vi "FPGA.vi"() -> ()   [LabVIEW 2016]
doc: "FPGA.vi\nv4.0c\nBuggy competition FPGA\n\nA Jackson 01/01/14"
uses:
  <vilib>/rvi/Emulation/niFpgaGetClockAttributes.vi
  <vilib>/rvi/Emulation/niFpgaSctlEmulationGetInTimedLoop.vi
  <vilib>/rvi/Emulation/niFpgaEmulationReportErrorSimple.vi
  <vilib>/rvi/Emulation/niFpgaProcessEmulError.vi
  <vilib>/rvi/eio/common/nirviEmuTemplateMethod_errors.vi
  <vilib>/rvi/Emulation/niFpgaCriticalErrorInLSC.vi
  <vilib>/eio/EIONode/EIONode.xnode
panel:
  in  "MS3":bool
  in  "MS2":bool
  in  "MS1":bool
  out "Motors Enabled":bool=TRUE
  in  "Motor 2 command":i8
  in  "Motor 1 command":i8
  out "Motor 2 Steps":i16
  out "Motor 1 Steps":i16
  in  "Motor Enable":bool
  in  "Step time":u32=100
  out "Potentiometer (V)":i16
  in  "Max sample interval (uS)":u32=62500
  in  "Measurement Width (Counts)":i64=4
  out "Enc 2 Interval (uS)":u32=10000000
  out "Enc 1 Interval (uS)":u32=10000000
  out "Encoder 2 dt (uS)":i64=-41
  out "Encoder 1 dt (uS)":i64=-41
  in  "Loop dT (uS)":u32=20
  out "Act. Loop uS":u32=20
  in  "Filter Iterations":i16=2
  in  "Reset encoder 1":bool
  out "Loop Count":i32=24102111
  out "Switch B (Blue)":bool
  out "Switch A (Green)":bool
  out "Encoder 2 Count":i64=-1
  out "Encoder 1 Count":i64=-1
  in  "Reset encoder 2":bool
  in  "stop":bool
  # "This FPGA VI will be controlled by the real-time VI and carries out low level hardware\n I/O via the FPGA part of the cRIO but it can also be used as a test panel for plotter hardware."
  # "Motors"
  # "Encoders"
  # "Timing"
  # "Microstepping"
  # "Switches"
  # "Potentiometer"
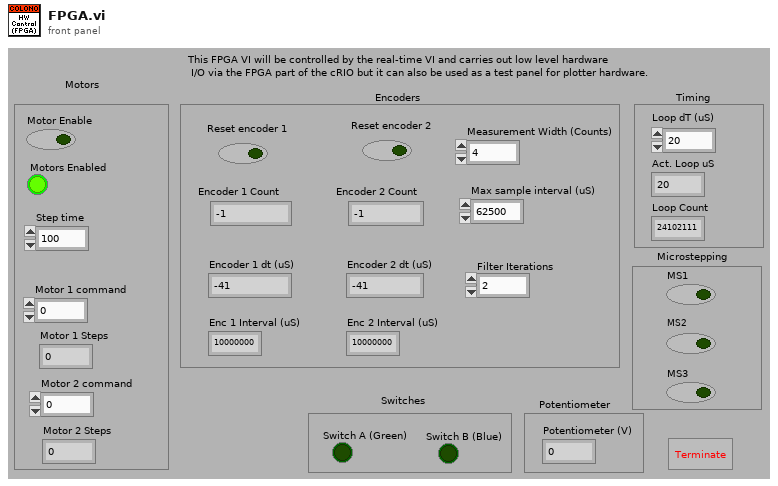
[diagram p1: front panel]
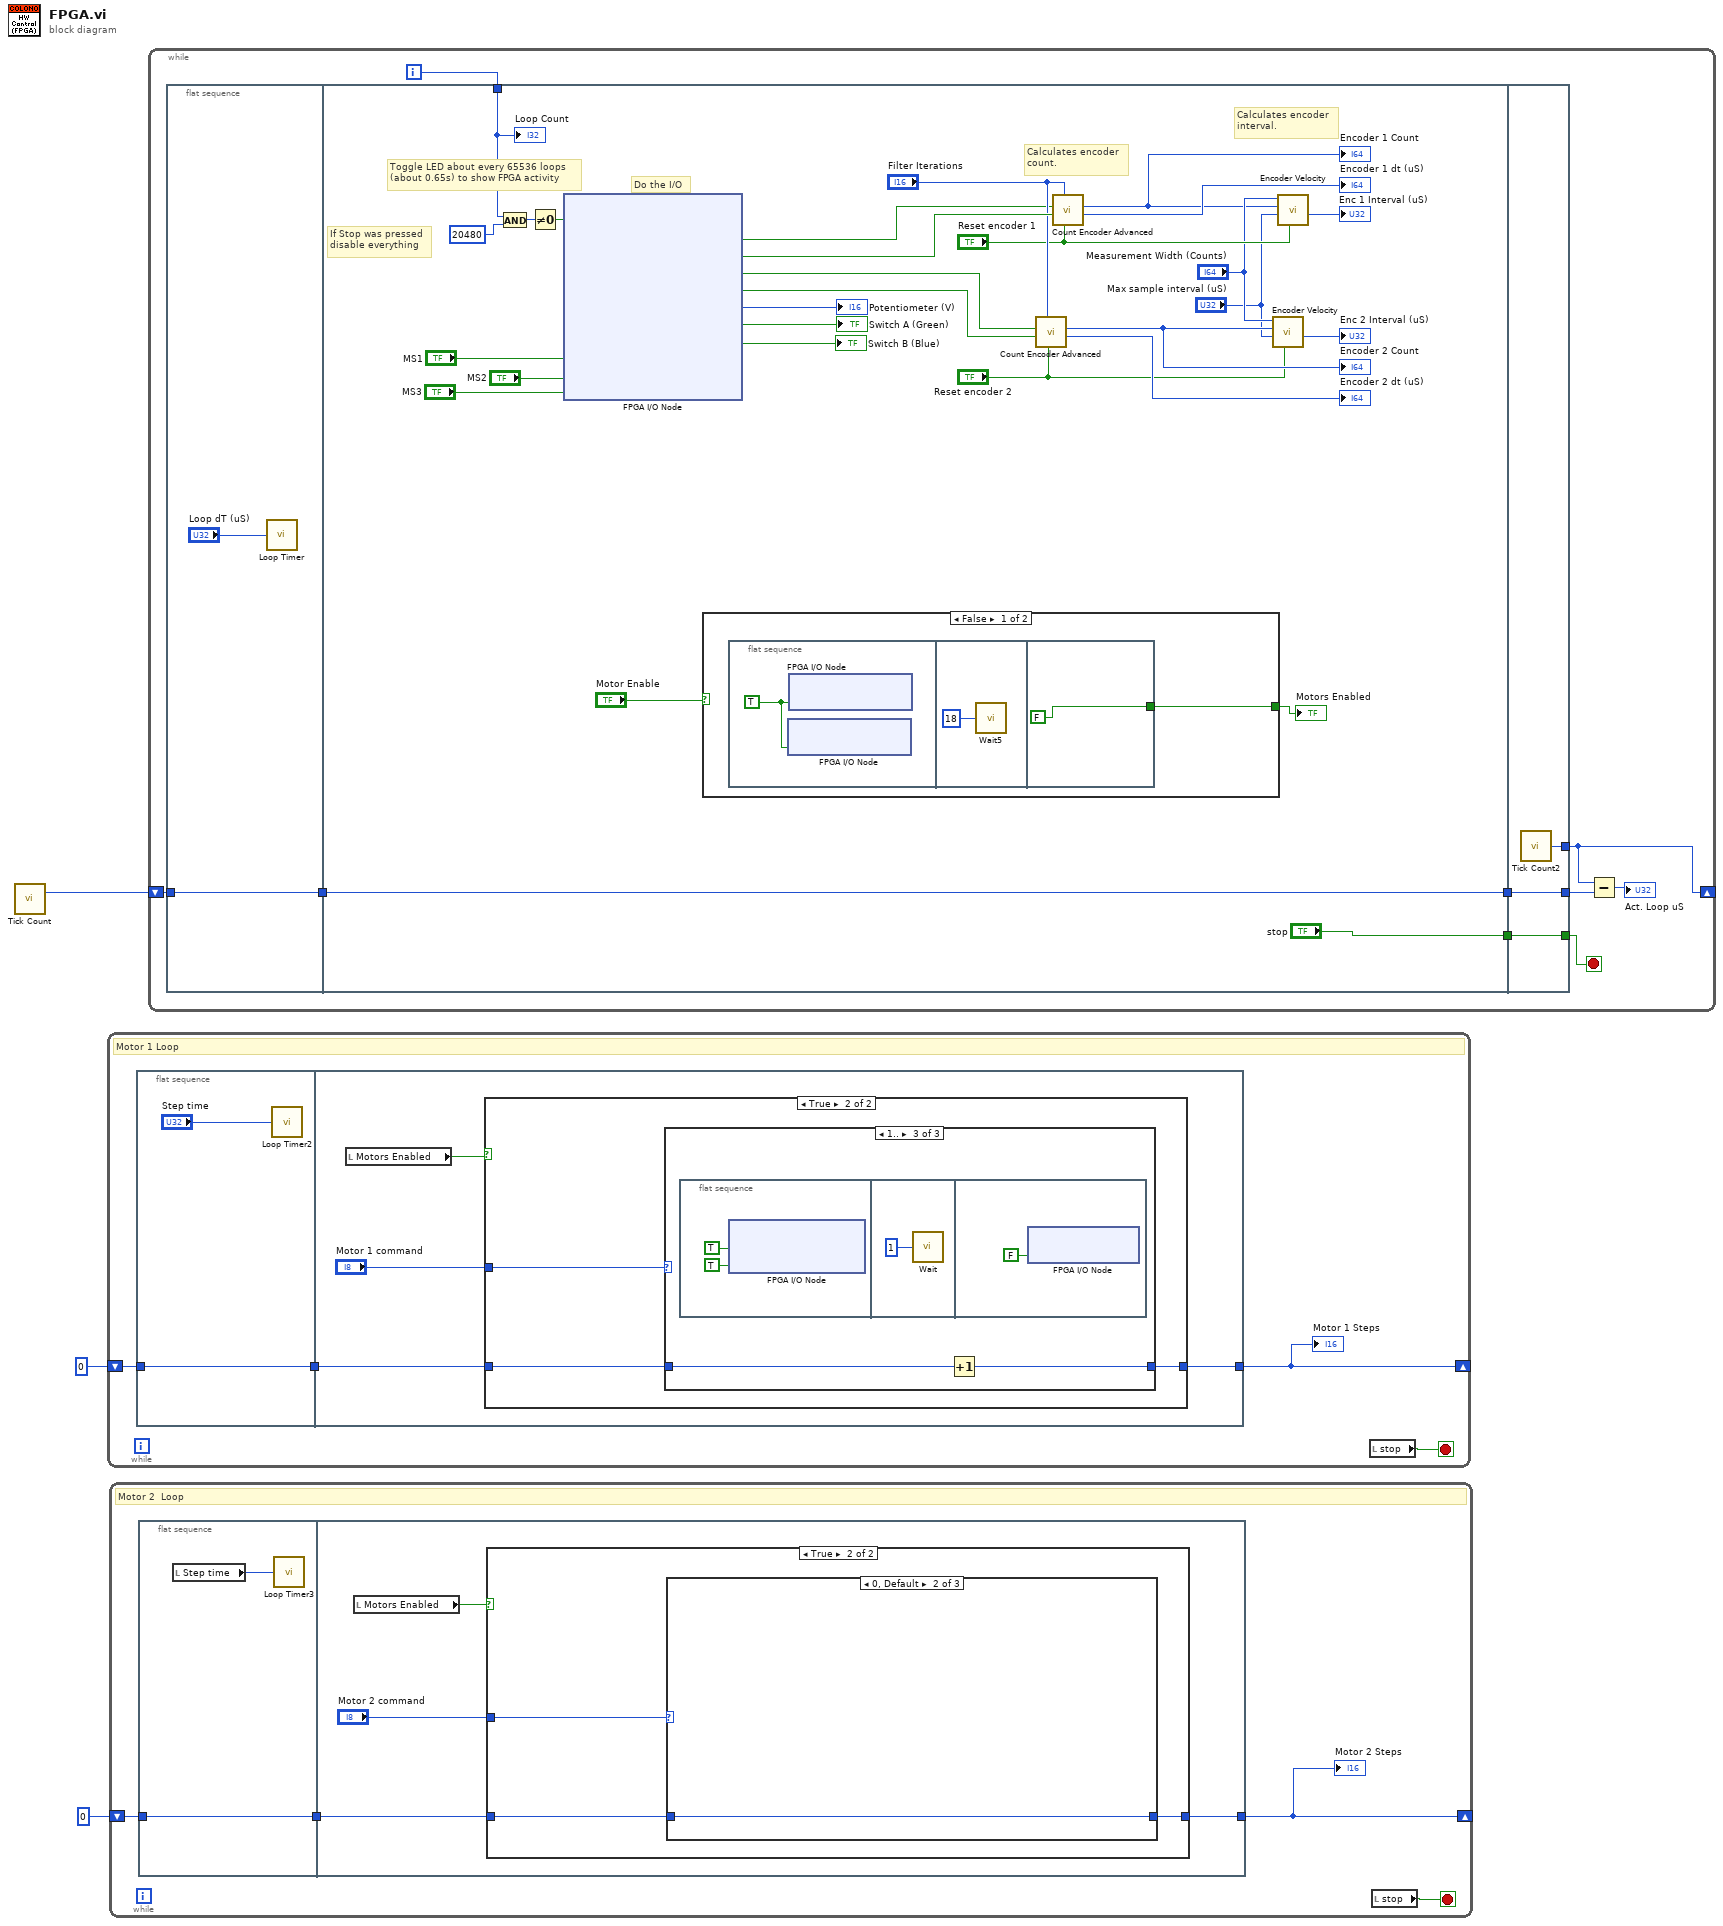
[diagram p0: block diagram]
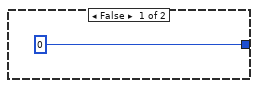
[diagram p2: hidden frame]
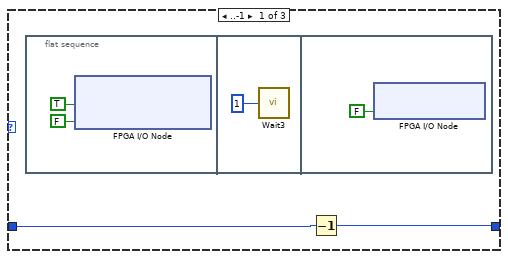
[diagram p3: hidden frame]
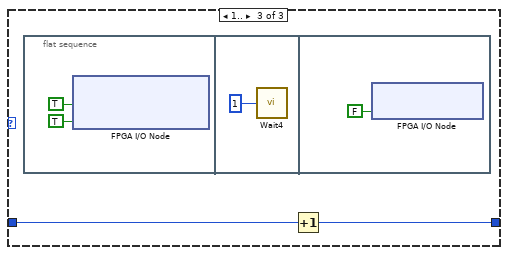
[diagram p4: hidden frame]
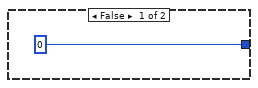
[diagram p5: hidden frame]
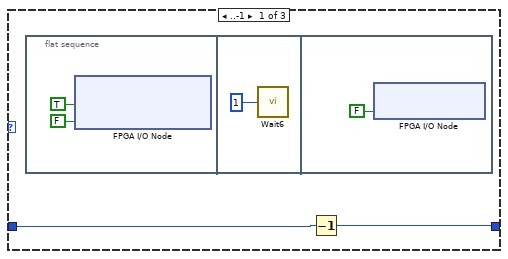
[diagram p6: hidden frame]
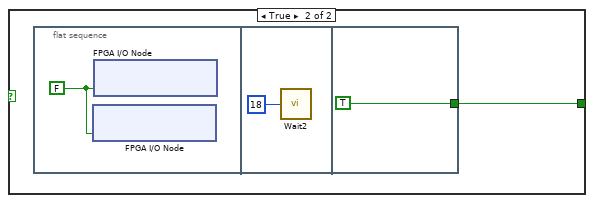
[diagram p8: hidden frame]
diagram:
  n1 = call "Tick Count"() -> ("Tick Count(uSec)"=w3:u32)
  n2 = while {
    shift-right: [w4] -> _
    shift-left: i16 0 -> [w5]
    stop <- w7 stop-if-true
    # "Motor 1 Loop"
    n3 = flat-sequence {
      tunnel: [w8] -> w6
      tunnel: w5 -> [w8]
      tunnel: [w13] -> w4
      tunnel: w6 -> [w11]
      frame #0 {
        n4 = call "Loop Timer2"("Count(mSec)"="Step time") -> ()  [unwired: 1 out]
      }
      frame #1 {
        n5 = local read "Motors Enabled"() -> (w10:bool)
        n6 = case shown="True" w10 {
          tunnel: w11 -> [_ w15]
          tunnel: [i16 0 w16] -> w13
          tunnel: "Motor 1 command" -> [_ w17]
          frame False {
          }
          frame True {
            n7 = case shown="1.." w17 {
              tunnel: [w18 w24 w25] -> w16
              tunnel: w15 -> [w19 w24 w26]
              frame ..-1 {
                n8 = flat-sequence {
                  frame #0 {
                    n9 = xnode "FPGA I/O Node"("Motor 1 Step"=TRUE ("Motor 1 A"), "Motor 1 Direction"=FALSE ("DIR0 Motor 1")) -> ()  [unwired: 2 in, 2 out]
                  }
                  frame #1 {
                    n10 = call "Wait6"("Count(mSec)"=u32 1) -> ()  [unwired: 1 out]
                  }
                  frame #2 {
                    n11 = xnode "FPGA I/O Node"("Motor 1 Step"=FALSE ("Motor 1 A")) -> ()  [unwired: 1 in, 1 out]
                  }
                }
                n12 = Decrement(x=w19) -> (x-1=w18:i16)
              }
              frame 0, Default {
              }
              frame 1.. {
                n13 = flat-sequence {
                  frame #0 {
                    n14 = xnode "FPGA I/O Node"("Motor 1 Step"=TRUE ("Motor 1 A"), "Motor 1 Direction"=TRUE ("DIR0 Motor 1")) -> ()  [unwired: 2 in, 2 out]
                  }
                  frame #1 {
                    n15 = call "Wait"("Count(mSec)"=u32 1) -> ()  [unwired: 1 out]
                  }
                  frame #2 {
                    n16 = xnode "FPGA I/O Node"("Motor 1 Step"=FALSE ("Motor 1 A")) -> ()  [unwired: 1 in, 1 out]
                  }
                }
                n17 = Increment(x=w26) -> (x+1=w25:i16)
              }
            }
          }
        }
      }
    }
    n18 = local read "stop"() -> (w7:bool)
    "Motor 1 Steps" <- w4
  }
  n19 = while {
    shift-right: [w31] -> _
    shift-left: i16 0 -> [w32]
    stop <- w34 stop-if-true
    # "Motor 2  Loop"
    n20 = flat-sequence {
      tunnel: [w36] -> w33
      tunnel: w32 -> [w36]
      tunnel: [w40] -> w31
      tunnel: w33 -> [w38]
      frame #0 {
        n21 = local read "Step time"() -> (w35:u32)
        n22 = call "Loop Timer3"("Count(mSec)"=w35) -> ()  [unwired: 1 out]
      }
      frame #1 {
        n23 = local read "Motors Enabled"() -> (w37:bool)
        n24 = case shown="True" w37 {
          tunnel: w38 -> [_ w42]
          tunnel: [i16 0 w43] -> w40
          tunnel: "Motor 2 command" -> [_ w44]
          frame False {
          }
          frame True {
            n25 = case shown="0, Default" w44 {
              tunnel: [w45 w51 w52] -> w43
              tunnel: w42 -> [w46 w51 w53]
              frame ..-1 {
                n26 = flat-sequence {
                  frame #0 {
                    n27 = xnode "FPGA I/O Node"("Motor 2 Step"=TRUE ("Motor 1 A"), "Motor 2 Direction"=FALSE ("DIR0 Motor 1")) -> ()  [unwired: 2 in, 2 out]
                  }
                  frame #1 {
                    n28 = call "Wait3"("Count(mSec)"=u32 1) -> ()  [unwired: 1 out]
                  }
                  frame #2 {
                    n29 = xnode "FPGA I/O Node"("Motor 2 Step"=FALSE ("Motor 1 A")) -> ()  [unwired: 1 in, 1 out]
                  }
                }
                n30 = Decrement(x=w46) -> (x-1=w45:i16)
              }
              frame 0, Default {
              }
              frame 1.. {
                n31 = flat-sequence {
                  frame #0 {
                    n32 = xnode "FPGA I/O Node"("Motor 2 Step"=TRUE ("Motor 1 A"), "Motor 2 Direction"=TRUE ("DIR0 Motor 1")) -> ()  [unwired: 2 in, 2 out]
                  }
                  frame #1 {
                    n33 = call "Wait4"("Count(mSec)"=u32 1) -> ()  [unwired: 1 out]
                  }
                  frame #2 {
                    n34 = xnode "FPGA I/O Node"("Motor 2 Step"=FALSE ("Motor 1 A")) -> ()  [unwired: 1 in, 1 out]
                  }
                }
                n35 = Increment(x=w53) -> (x+1=w52:i16)
              }
            }
          }
        }
      }
    }
    n36 = local read "stop"() -> (w34:bool)
    "Motor 2 Steps" <- w31
  }
  n37 = while {
    shift-right: [w60] -> _
    shift-left: w3 -> [w66]
    i -> [w59]
    stop <- w58 stop-if-true
    n38 = flat-sequence {
      tunnel: w66 -> [w68]
      tunnel: [w68] -> w65
      tunnel: w65 -> [w81]
      tunnel: ["stop"] -> w62
      tunnel: [w81] -> w61
      tunnel: w59 -> [w80]
      tunnel: [w107] -> w63
      tunnel: [w108] -> w58
      tunnel: w62 -> [w108]
      tunnel: w61 -> [w107]
      tunnel: [w106] -> w60
      frame #0 {
        n39 = call "Loop Timer"("Count(uSec)"="Loop dT (uS)") -> ()  [unwired: 1 out]
      }
      frame #1 {
        # "Calculates encoder\ninterval."
        # "Calculates encoder\ncount."
        # "Toggle LED about every 65536 loops\n(about 0.65s) to show FPGA activity"
        # "If Stop was pressed\ndisable everything"
        # "Do the I/O"
        n40 = And(x=w80, y=20480) -> (x .and. y?=w92:i32)
        n41 = Not Equal To 0?(x=w92) -> (x != 0?=w82:bool)
        n42 = xnode "FPGA I/O Node"("FPGA Working"=w82, "MS1"="MS1", "MS2"="MS2", "MS3"="MS3") -> ("Motor 1/Encoder Phase A"=w79:bool, "Motor 1/Encoder Phase B"=w97:bool, "Motor 2/Encoder Phase A"=w95:bool, "Motor 2/Encoder Phase B"=w94:bool, "Potentiometer"=→"Potentiometer (V)":i16, "Switch 1 - Green"=→"Switch A (Green)":bool, "Switch 2 - Black"=→"Switch B (Blue)":bool)  [unwired: 11 in, 11 out]
        n43 = case shown="False" "Motor Enable" {
          tunnel: [w98 w102] -> w73
          frame False {
            n44 = flat-sequence {
              tunnel: [FALSE ("Motors Enabled")] -> w98
              frame #0 {
                w99 = TRUE ("Motor 1 A")
                n45 = xnode "FPGA I/O Node"("Motor 2 Enable"=w99) -> ()  [unwired: 1 in, 1 out]
                n46 = xnode "FPGA I/O Node"("Motor 1 Enable"=w99) -> ()  [unwired: 1 in, 1 out]
              }
              frame #1 {
                n47 = call "Wait5"("Count(uSec)"=u32 18 ("Count(mSec)")) -> ()  [unwired: 1 out]
              }
              frame #2 {
              }
            }
          }
          frame True {
            n48 = flat-sequence {
              tunnel: [TRUE ("Motors Enabled")] -> w102
              frame #0 {
                w103 = FALSE ("Motor 1 A")
                n49 = xnode "FPGA I/O Node"("Motor 2 Enable"=w103) -> ()  [unwired: 1 in, 1 out]
                n50 = xnode "FPGA I/O Node"("Motor 1 Enable"=w103) -> ()  [unwired: 1 in, 1 out]
              }
              frame #1 {
                n51 = call "Wait2"("Count(uSec)"=u32 18 ("Count(mSec)")) -> ()  [unwired: 1 out]
              }
              frame #2 {
              }
            }
          }
        }
        "Motors Enabled" <- w73
        n52 = call "Count Encoder Advanced.vi"("Initialise"="Reset encoder 2", "Filter Iterations"="Filter Iterations", "Encoder B Signal In"=w94, "Encoder A Signal In"=w95) -> ("dt (uS)"=→"Encoder 2 dt (uS)":i64, "Encoder Count Out"=w89:i64)  [unwired: 6 in]
        "Encoder 2 Count" <- w89
        n53 = call "Count Encoder Advanced.vi"("Initialise"="Reset encoder 1", "Filter Iterations"="Filter Iterations", "Encoder B Signal In"=w97, "Encoder A Signal In"=w79) -> ("dt (uS)"=→"Encoder 1 dt (uS)":i64, "Encoder Count Out"=w78:i64)  [unwired: 6 in]
        "Encoder 1 Count" <- w78
        n54 = call "Encoder Velocity.vi"("Initialize?"="Reset encoder 2", "Max sample interval (uS)"="Max sample interval (uS)", "Encoder Count In"=w89, "Measurement Width (Counts)"="Measurement Width (Counts)") -> ("Enc Interval (uS)"=→"Enc 2 Interval (uS)":u32)  [unwired: 6 in, 1 out]
        n55 = call "Encoder Velocity.vi"("Initialize?"="Reset encoder 1", "Max sample interval (uS)"="Max sample interval (uS)", "Encoder Count In"=w78, "Measurement Width (Counts)"="Measurement Width (Counts)") -> ("Enc Interval (uS)"=→"Enc 1 Interval (uS)":u32)  [unwired: 6 in, 1 out]
        "Loop Count" <- w80
      }
      frame #2 {
        n56 = call "Tick Count2"() -> ("Tick Count(uSec)"=w106:u32)
      }
    }
    n57 = Subtract(x=w60, y=w63) -> (x-y=→"Act. Loop uS":u32)
  }
